vi "Drop Message Core.vi"(11 "Lock Publication Msg in":refnum<class "Lock Publication Msg.lvclass">) -> ()   [LabVIEW 2019, in "IMediator.lvlib" / "Lock Publication Msg.lvclass"]
doc: "(<B>Filename</B>: Actor Framework.lvlib:Message.lvclass:Drop Message Core.vi)\n\nDefines what a message does if it is in the message queue when the queue is released. At this point, the actor has shut down, so it will never process the message.\n\nBy default, this method does nothing. A child class may override it to define behavior. National Instruments provides the Reply Msg class to override this method. This class releases its internal queue, which causes any caller of the Send Message and Wait For Response method to stop waiting and return an error."
uses:
  <vilib>/gpm_packages/@cs/mva-core/Source/IMediator/IMediator Messages/Lock Publication Msg/Lock Publication Msg.lvclass
  <vilib>/gpm_packages/@cs/mva-core/Source/IMediator/IMediator Messages/Lock Publication Msg/Lock Publication Msg.lvclass/Lock Publication Msg.ctl
  <vilib>/Utility/error.llb/Error Cluster From Error Code.vi
  <vilib>/ErrorRing/Error Ring.xnode
  <vilib>/gpm_packages/@cs/transport/Source/ITransport/ITransport.lvclass
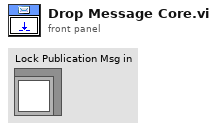
[diagram p1: front panel]
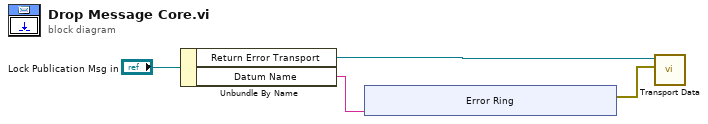
[diagram p0: block diagram]
diagram:
  n1 = Unbundle By Name("Lock Publication Msg in") -> ("Return Error Transport"=w3:refnum<class "ITransport.lvclass">, "Datum Name"=w1:string)
  n2 = xnode "Error Ring"("parameter 0"=w1) -> ("error out"=w2:errorcluster)
  n3 = call <vilib>:"Transport Data.vi"("Value"=w2, "ITransport in"=w3) -> ()  [unwired: 8 in, 2 out]
